vi "Read 1 Swipe Vector.vi"(8 "Error In":errorcluster, 11 "Leap Handle 2":T2) -> (0 "Error Out":errorcluster, 1 "Gesture State":T1, 2 "Swipe Vector":cluster{"X":sgl, "Y":sgl, "Z":sgl}, 3 "Leap Handle":T2)   [LabVIEW 2011, in "LVH-Leap.lvlib"]
doc: "Read one swipe gesture vector."
uses:
  LVH-Leap.lvlib
  Private/Type Defs/Leap Handle.ctl
  C:/github/labviewhacker/LVH-Leap/LabVIEW/vi.lib/LabVIEW Hacker/Leap/Private/Libs/LeapCSharp.NET3.5.dll
  Private/Libs/LeapCSharp.NET3.5.dll
  Private/Type Defs/Gesture State.ctl
  Read N Swipes.vi
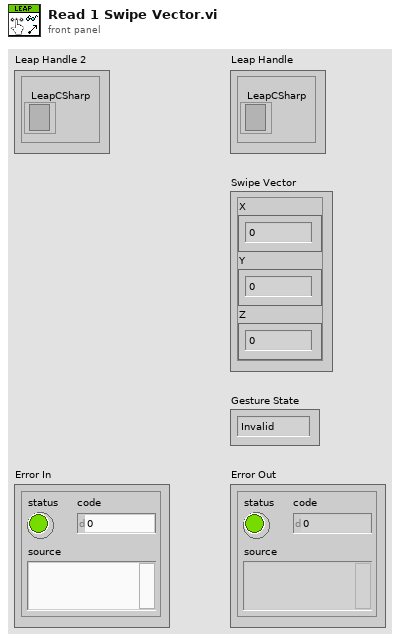
[diagram p1: front panel]
types:
  T1 = typedef "LVH-Leap.lvlib/Gesture State.ctl" = enum16{"Invalid", "Start", "Update", "Stop"}
  T2 = typedef "LVH-Leap.lvlib/Leap Handle.ctl" = cluster{"LeapCSharp":refnum<k24>}
  T3 = typedef "LVH-Leap.lvlib/Gesture Swipe.ctl" = cluster{"Common":T4, "Direction":T6, "Position":T6, "Start Position":T6, "Speed":dbl}
  T4 = typedef "LVH-Leap.lvlib/Gesture Common.ctl" = cluster{"ID":dbl, "Duration (S)":dbl, "Gesture Type":T5, "Gesture State":T1}
  T5 = typedef "LVH-Leap.lvlib/Gesture Type.ctl" = enum16{"Invalid", "Swipe", "Circle", "Screen Tap", "Key Tap"}
  T6 = typedef "LVH-Leap.lvlib/Vector.ctl" = cluster{"Pitch":sgl, "Yaw":sgl, "Roll":sgl, "Magnitude":sgl, "XYZ":sgl[]}
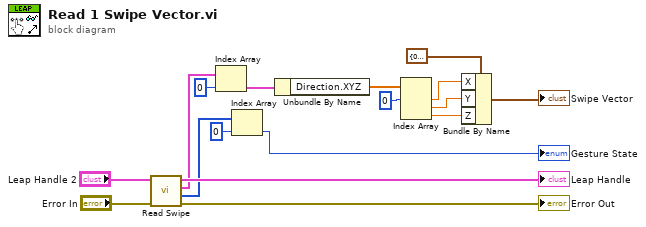
[diagram p0: block diagram]
diagram:
  n1 = call-poly "Read Swipe.vi"("Error In"="Error In", "Leap Handle"="Leap Handle 2") -> ("Error Out"=→"Error Out":errorcluster, "Swipe Statuses"=w3:T1[], "Swipe Gestures"=w7:T3[], "Leap Handle"=→"Leap Handle":T2)  [unwired: 6 in]
  n2 = Index Array(array=w7, index=0) -> (element=w6:T3)
  n3 = Index Array(array=w3, index=0) -> (element=→"Gesture State":T1)
  n4 = Unbundle By Name(w6) -> ("Direction.XYZ"=w12:sgl[])
  n5 = Index Array(array=w12, index #1=0 ("index")) -> (element #1=w10:sgl, element #2=w9:sgl, element #3=w8:sgl)  [unwired: 2 in]
  n6 = Bundle By Name(cluster=cluster{"X":sgl, "Y":sgl, "Z":sgl} {"X"=0.0, "Y"=0.0, "Z"=0.0} ("element"), "X"=w10, "Y"=w9, "Z"=w8) -> (→"Swipe Vector":cluster{"X":sgl, "Y":sgl, "Z":sgl})
